vi "Write UEGO.vi"(8 "error in (no error)":errorcluster, 9 "RT UEGO Settling Time Data in":T1, 10 "UEGO Engine Refs in":T2 {"RT IDs"."Slot #" max=15; "RT IDs"."Chip Address (A2 A1 A0)" max=7; "RT Block Data Refs"."Data Reference" format="%.0x"}, 11 "DMA FIFO Ref in":refnum<k20>) -> (0 "error out":errorcluster, 1 "RT UEGO Settling Time Data out":T1, 2 "UEGO Engine Refs out":T2 {"RT IDs"."Slot #" max=15; "RT IDs"."Chip Address (A2 A1 A0)" max=7; "RT Block Data Refs"."Data Reference" format="%.0x"})   [LabVIEW 2014, in "SLSC configuration Engine.lvlib"]
uses:
  SLSC configuration Engine.lvlib
  Type Defs/RT Engine Refs.ctl
  Shared/Type Defs/RT IDs.ctl
  Shared/SPI Utility/Slot #.ctl
  Shared/MCP23S17/Chip Address.ctl
  <vilib>/NI Veristand/Custom Device API/Block Data Reference.ctl
  <vilib>/NI Veristand/Custom Device API/Data Reference.ctl
  Type Defs/RT UEGO Setting Time Data.ctl
  <vilib>/NI Veristand/Custom Device API/Global Data Refs.vi
  Shared/Constants.vi
  <vilib>/NI Veristand/Custom Device API/Custom Device API.lvlib
  Shared/SLSC configuration Shared.lvlib
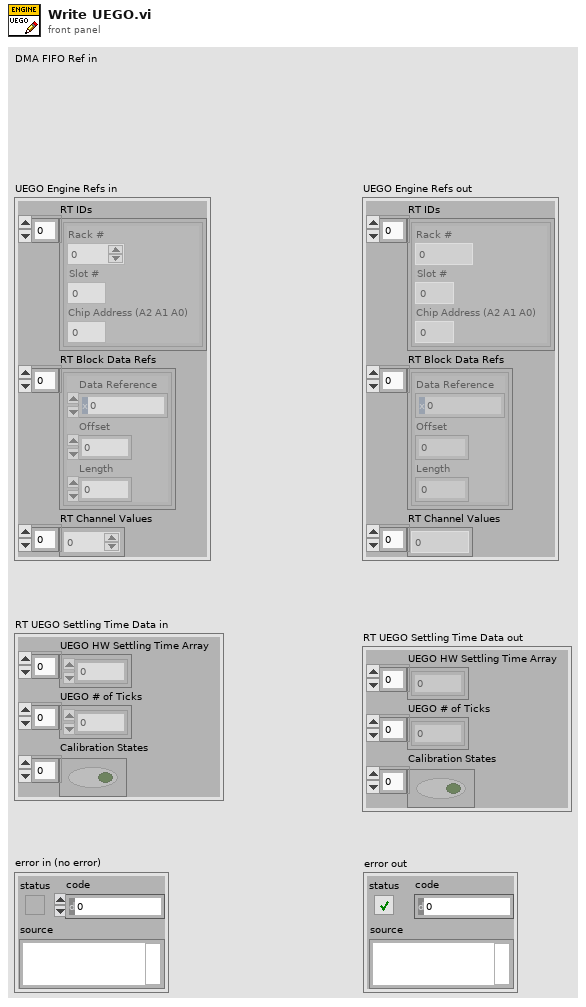
[diagram p1: front panel]
types:
  T1 = typedef "SLSC configuration Engine.lvlib/RT UEGO Setting Time Data.ctl" = cluster{"UEGO HW Settling Time Array":u32[], "UEGO # of Ticks":u32[], "Calibration States":bool[]}
  T2 = typedef "SLSC configuration Engine.lvlib/RT Engine Refs.ctl" = cluster{"RT IDs":T3[], "RT Block Data Refs":T6[], "RT Channel Values":dbl[]}
  T3 = typedef "SLSC configuration Shared.lvlib/RT IDs.ctl" = cluster{"Rack #":u8, "Slot #":T4, "Chip Address (A2 A1 A0)":T5}
  T4 = typedef "SLSC configuration Shared.lvlib/Slot #.ctl" = u8
  T5 = typedef "SLSC configuration Shared.lvlib/Chip Address.ctl" = u8
  T6 = typedef "Custom Device API.lvlib/Block Data Reference.ctl" = cluster{"Data Reference":T7, "Offset":i32, "Length":i32}
  T7 = typedef "Custom Device API.lvlib/Data Reference.ctl" = i32
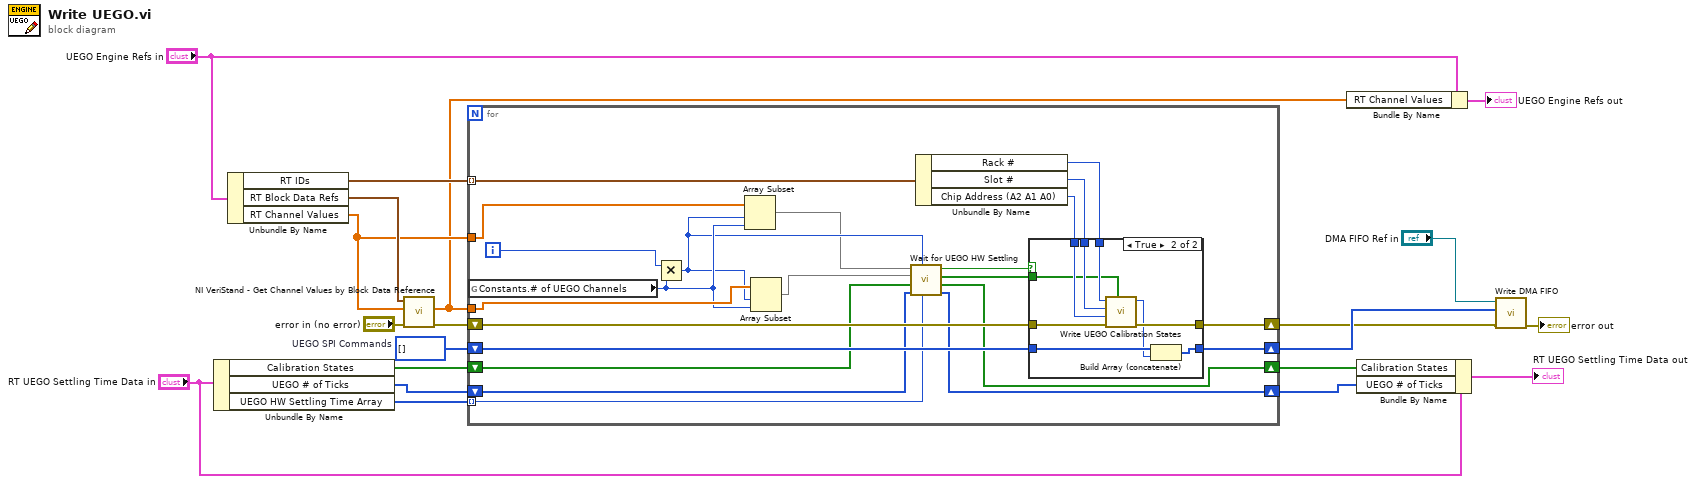
[diagram p0: block diagram]
diagram:
  w12 = u64[] []  # UEGO SPI Commands
  n1 = Unbundle By Name("RT UEGO Settling Time Data in") -> ("Calibration States"=w2:bool[], "UEGO # of Ticks"=w7:u32[], "UEGO HW Settling Time Array"=w3:u32[])
  n2 = Unbundle By Name("UEGO Engine Refs in") -> ("RT IDs"=w17:T3[], "RT Block Data Refs"=w20:T6[], "RT Channel Values"=w15:dbl[])
  n3 = call <vilib>:"NI VeriStand - Get Channel Values by Block Data Reference.vi"("error in (no error)"="error in (no error)", "Values Array in"=w15, "Block Data Ref"=w20) -> ("error out"=w18:errorcluster, "Values Array out"=w14:dbl[])  [unwired: 6 in, 1 out]
  n4 = for {
    shift-right: [w40] -> w9
    shift-left: w18 -> [w41]
    tunnel: w17 -> [w42] mode=indexing
    tunnel: w14 -> [w35]
    tunnel: w15 -> [w37]
    shift-right: [w38] -> w10
    shift-left: w12 -> [w39]
    shift-right: [w29] -> w5
    shift-left: w7 -> [w30]
    tunnel: w3 -> [w25] mode=indexing
    shift-right: [w21] -> w1
    shift-left: w2 -> [w24]
    i -> [w36]
    n5 = global read "Constants.vi" "Constants.# of UEGO Channels"() -> (w34:u8)
    n6 = Multiply(x=w36, y=w34) -> (x*y=w28:i32)
    n7 = Array Subset(array=w37, index=w28, length=w34) -> (w27:dbl[])
    n8 = Array Subset(array=w35, index=w28, length=w34) -> (w26:dbl[])
    n9 = call "Wait for UEGO HW Settling.vi"("HW Settling Time Ticks"=w25, "Starting Index"=w28, "Current Tick Count in"=w30, "Prev States"=w24, "Current Values"=w26, "Previous Values"=w27) -> ("Current Tick Count out"=w29:u32[], "Current States"=w21:bool[], "New State"=w22:bool[], "Update State?"=w23:bool)  [unwired: 2 in]
    n10 = Unbundle By Name(w42) -> ("Rack #"=w32:u8, "Slot #"=w31:T4, "Chip Address (A2 A1 A0)"=w33:T5)
    n11 = case shown="True" w23 {
      tunnel: w41 -> [w44 w53]
      tunnel: [w44 w52] -> w40
      tunnel: w39 -> [w43 w51]
      tunnel: [w43 w50] -> w38
      tunnel: w33 -> [_ w49]
      tunnel: w32 -> [_ w47]
      tunnel: w31 -> [_ w46]
      tunnel: w22 -> [_ w45]
      frame False {
      }
      frame True {
        n12 = call "Write UEGO Calibration States.vi"("UEGO Calibration States"=w45, "error in (no error)"=w53, "Chip Address (A2 A1 A0)"=w49, "Slot #"=w46, "Rack #"=w47) -> ("error out"=w52:errorcluster, "FIFO SPI Message"=w48:u64)  [unwired: 4 in, 1 out]
        n13 = Build Array (concatenate)(w51, w48) -> (w50:u64[])
      }
    }
  }
  n14 = Bundle By Name(cluster="UEGO Engine Refs in", "RT Channel Values"=w14) -> (→"UEGO Engine Refs out":T2)
  n15 = Bundle By Name(cluster="RT UEGO Settling Time Data in", "Calibration States"=w1, "UEGO # of Ticks"=w5) -> (→"RT UEGO Settling Time Data out":T1)
  n16 = call "Write DMA FIFO.vi"("error in (no error)"=w9, "FIU SPI Commands"=w10, "DMA FIFO Ref in"="DMA FIFO Ref in") -> ("error out"=→"error out":errorcluster)  [unwired: 8 in]
